vi "beginKickoffEnemyPlayVSS.vi"(8 "error in (no error)":errorcluster, 9 "FoulVSS":T1=enum."PENALTY_KICK_ENEMY", 10 "queue 2":T2(array[ring]), 11 "KickoffEnemyPlayVSS in":refnum<class "KickoffEnemyPlayVSS.lvclass">) -> (0 "error out":errorcluster, 2 "logical AND":bool, 3 "KickoffEnemyPlayVSS out":refnum<class "KickoffEnemyPlayVSS.lvclass">)   [LabVIEW 2023, in "KickoffEnemyPlayVSS.lvclass"]
uses:
  KickoffEnemyPlayVSS.lvclass
  Command.ctl
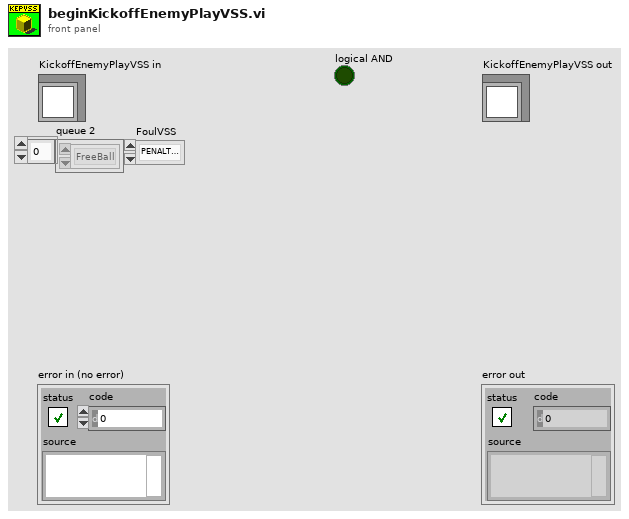
[diagram p1: front panel]
types:
  T1 = typedef "Command.ctl" = enum16{"AUTO", "GAME_ON", "STOP", "HALT", "KICKOFF_ALLY", "KICKOFF_ENEMY", "FREE_BALL", "GOAL_KICK_ENEMY", "GOAL_KICK_ALLY", "PENALTY_KICK_ENEMY", "PENALTY_KICK_ALLY", "FREE_KICK"}
  T2 = enum16{"FreeBall", "PrepareFreeBall", "GoalKickEnemy", "GoalKickAlly", "KickoffAlly", "KickoffEnemy", "PrepareGoalKickEnemy", "PrepareGoalKickAlly", "Stop", "PrepareKickoffEnemy", "PrepareKickoffAlly", "PreparePenaltyEnemy", "Timeout", "DeadBall", "NormalGame", "KickPenaltyAlly", "PenaltyEnemy", "BallChallenge", "PreparePenaltyAlly", "Halt"}[]
  T3 = enum16{"FreeBall", "PrepareFreeBall", "GoalKickEnemy", "GoalKickAlly", "KickoffAlly", "KickoffEnemy", "PrepareGoalKickEnemy", "PrepareGoalKickAlly", "Stop", "PrepareKickoffEnemy", "PrepareKickoffAlly", "PreparePenaltyEnemy", "Timeout", "DeadBall", "NormalGame", "KickPenaltyAlly", "PenaltyEnemy", "BallChallenge", "PreparePenaltyAlly", "Halt"}
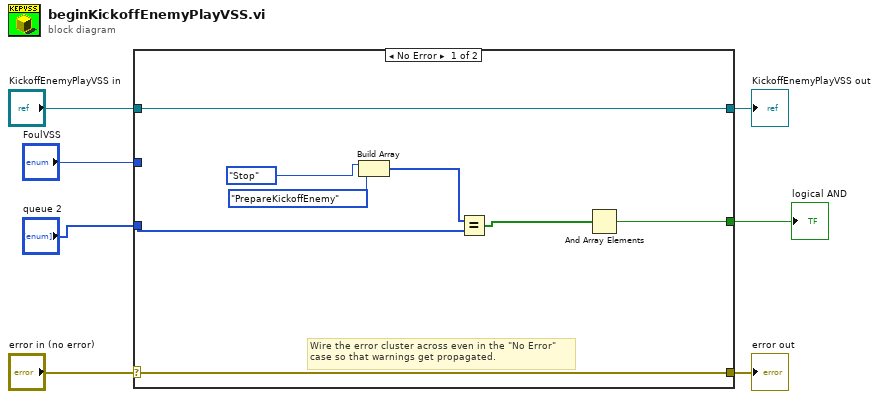
[diagram p0: block diagram]
diagram:
  n1 = case shown="No Error" "error in (no error)" {
    selector: "error in (no error)" -> [w14 w17]
    tunnel: [w14 w17] -> w6
    tunnel: [w15 w16] -> w4
    tunnel: "KickoffEnemyPlayVSS in" -> [w15 w16]
    tunnel: "queue 2" -> [w10 _]
    tunnel: "FoulVSS" -> [_ _]
    tunnel: [w8 _] -> w1
    frame No Error {
      # "Wire the error cluster across even in the \"No Error\"\ncase so that warnings get propagated."
      n2 = Build Array(T3."Stop" ("VssPlay"), T3."PrepareKickoffEnemy" ("VssPlay")) -> (w11:T2)
      n3 = Equal?(x=w11, y=w10) -> (x = y?=w9:bool[])
      n4 = And Array Elements(Boolean array=w9) -> (logical AND=w8:bool)
    }
    frame Error {
    }
  }
  "error out" <- w6
  "KickoffEnemyPlayVSS out" <- w4
  "logical AND" <- w1
